vi "array.vi"(0 "x":dbl, 1 "y":dbl, 3 "array":dbl[](array[numeric])) -> (7 "appended array":dbl[](array[numeric]))   [LabVIEW 2014]
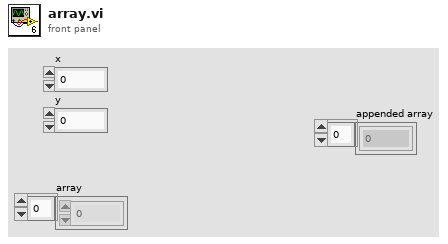
[diagram p1: front panel]
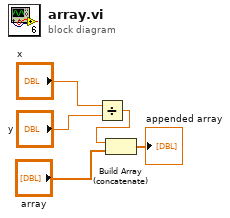
[diagram p0: block diagram]
diagram:
  n1 = Divide(x="x", y="y") -> (x/y=w5:dbl)
  n2 = Build Array (concatenate)(w5, "array") -> (→"appended array":dbl[])
